vi "Ion.vi"() -> (1 "Ion (ppm)":dbl format="%.2f")   [LabVIEW 2016]
uses:
  Kpro Globals.vi
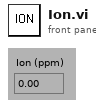
[diagram p1: front panel]
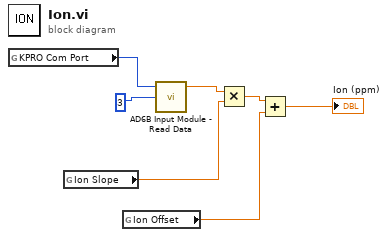
[diagram p0: block diagram]
diagram:
  n1 = global read "Kpro Globals.vi" "KPRO Com Port"() -> (w3:i32)
  n2 = global read "Kpro Globals.vi" "Ion Slope"() -> (w1:dbl)
  n3 = global read "Kpro Globals.vi" "Ion Offset"() -> (w2:dbl)
  n4 = call "AD6B Input Module - Read Data.VI"("address (0 to 255)"=3, "port number (1:com2)"=w3) -> ("scaled data"=w6:dbl)  [unwired: 1 in, 2 out]
  n5 = Multiply(x=w6, y=w1) -> (x*y=w5:dbl)
  n6 = Add(x=w5, y=w2) -> (x+y=→"Ion (ppm)":dbl)
